vi "Trial 4 A4.vi"() -> ()   [LabVIEW 2022 SP3]
uses:
  Documents/Control 1 Trial 3.ctl
panel:
  out "Time remaining":i32
  in  "Start":bool
  in  "Stop":bool
  in  "Washing Mode Menu":T1(ring)
  out "Washing Stage":string
  out "Washing Mode":string
  in  "On/Off":bool
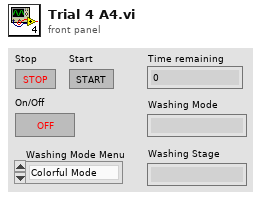
[diagram p1: front panel]
types:
  T1 = enum16{"Colorful Mode", "Intensive Mode", "Quick Wash"}
  T2 = typedef "Control 1 Trial 3.ctl" = enum16{"Off", "On", "Start Washing", "Pre-rinse", "Main Washing", "Final Spin", "Done Washing"}
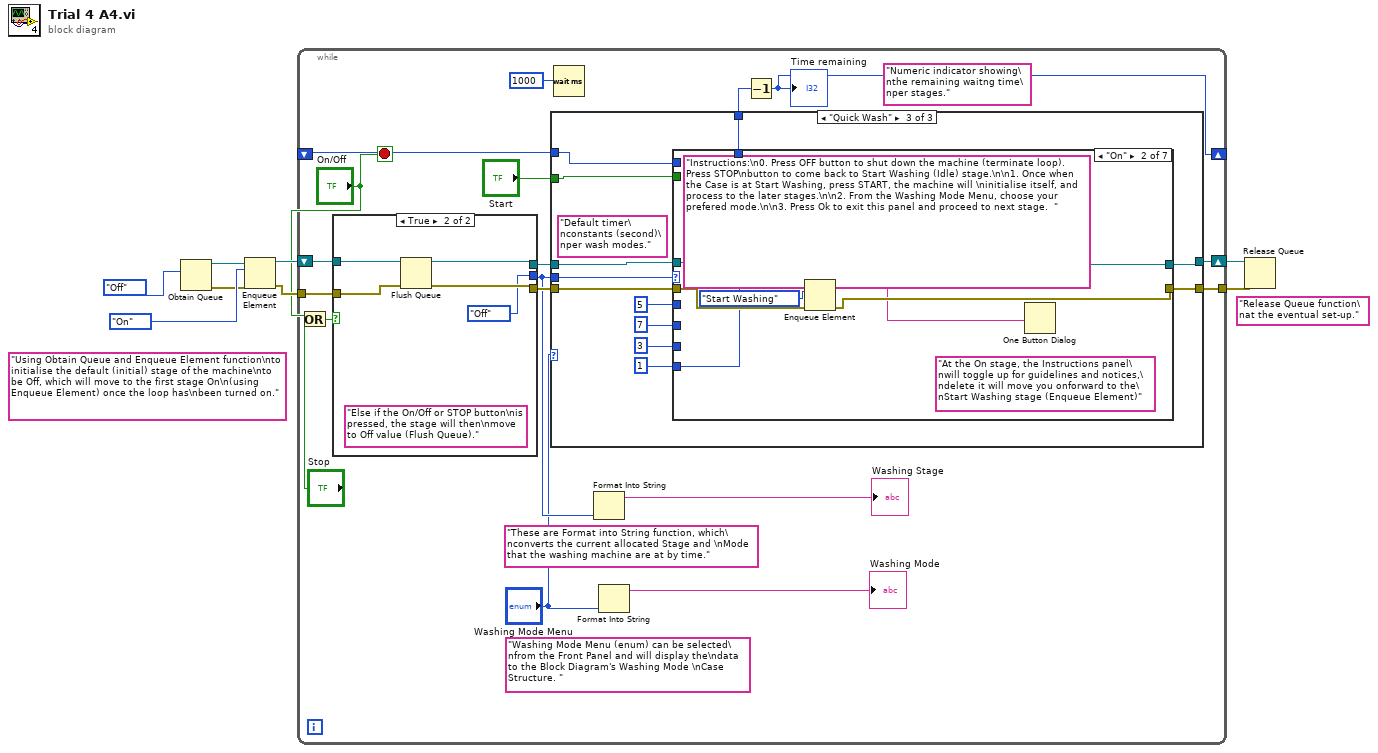
[diagram p0: block diagram]
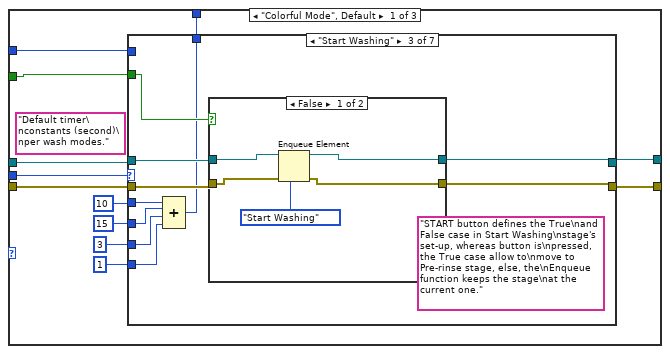
[diagram p2: hidden frame]
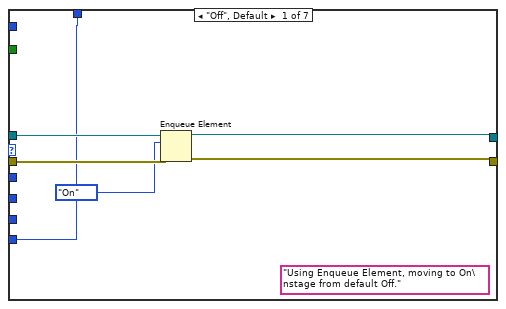
[diagram p3: hidden frame]
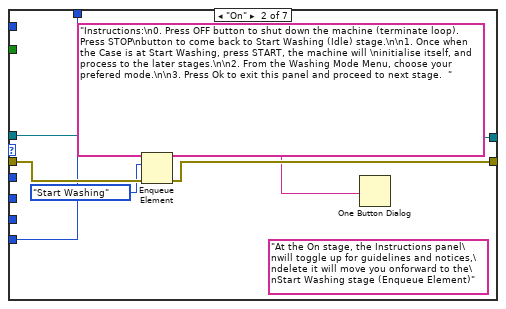
[diagram p4: hidden frame]
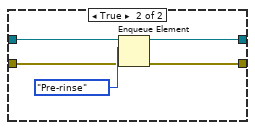
[diagram p5: hidden frame]
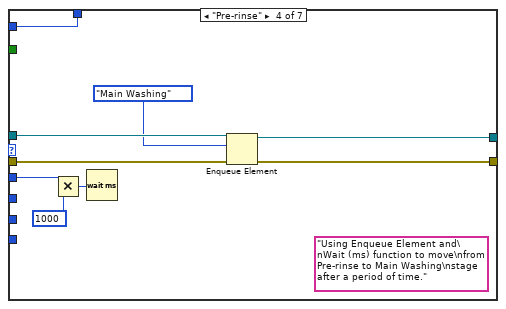
[diagram p6: hidden frame]
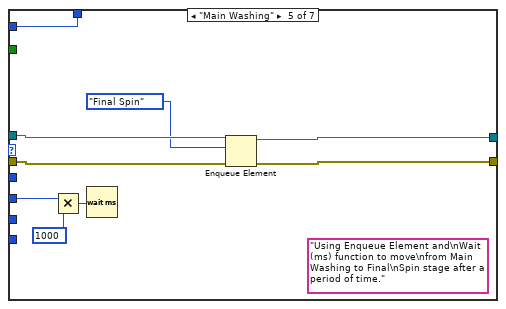
[diagram p7: hidden frame]
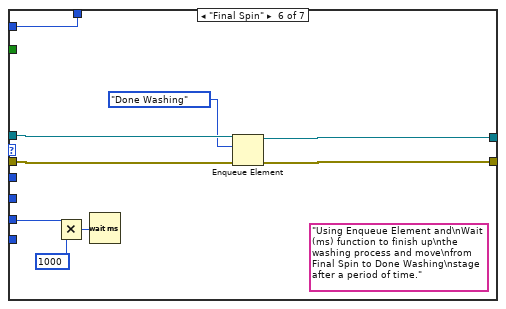
[diagram p8: hidden frame]
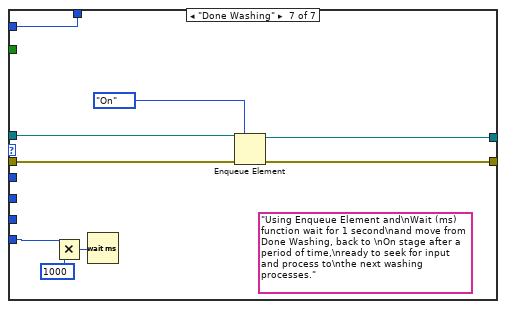
[diagram p9: hidden frame]
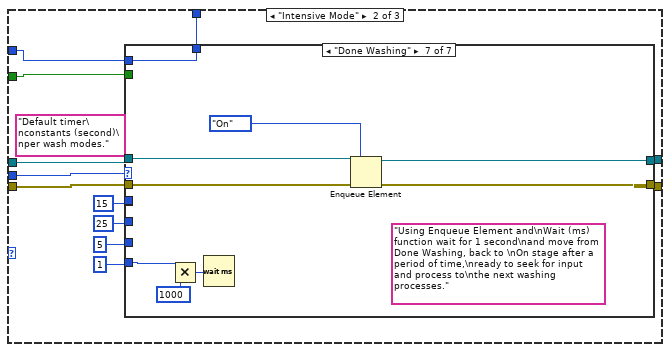
[diagram p10: hidden frame]
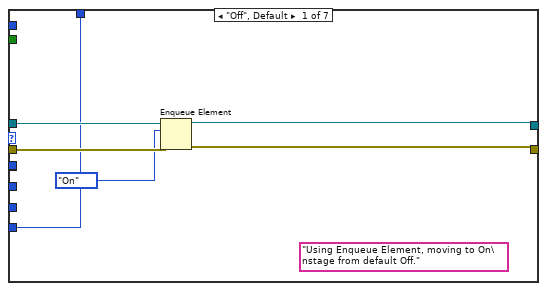
[diagram p11: hidden frame]
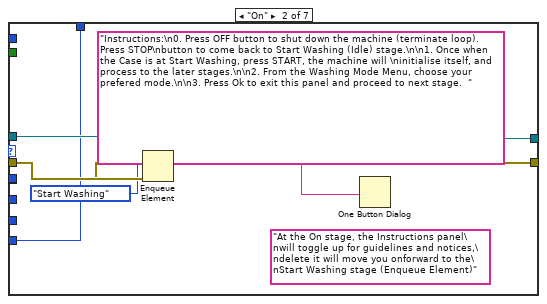
[diagram p12: hidden frame]
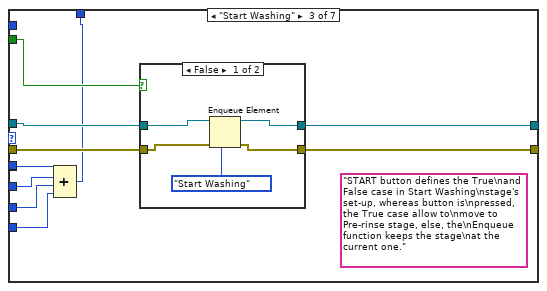
[diagram p13: hidden frame]
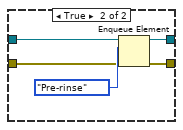
[diagram p14: hidden frame]
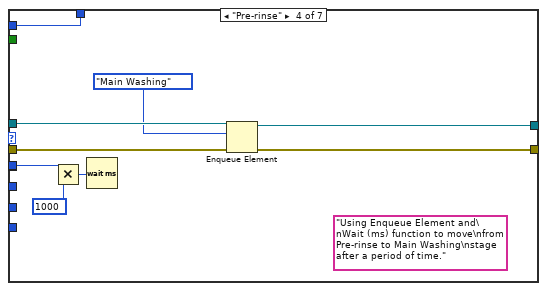
[diagram p15: hidden frame]
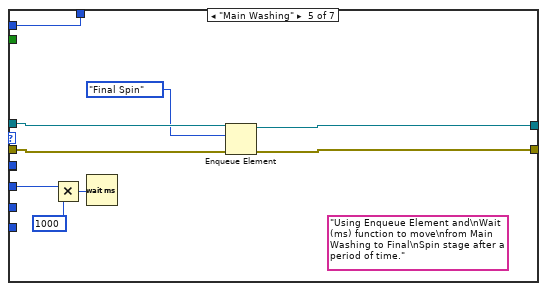
[diagram p16: hidden frame]
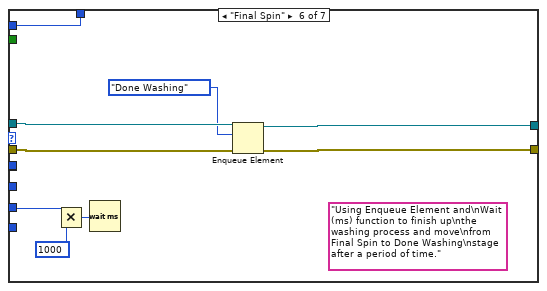
[diagram p17: hidden frame]
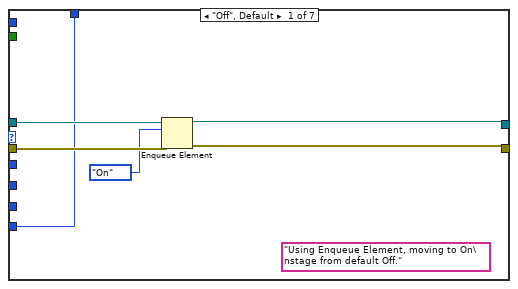
[diagram p18: hidden frame]
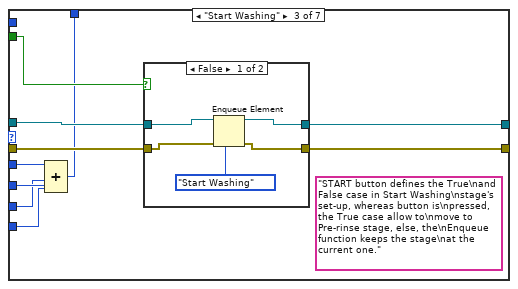
[diagram p19: hidden frame]
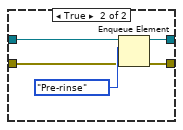
[diagram p20: hidden frame]
diagram:
  (unwired) "Release Queue function\nat the eventual set-up."
  (unwired) "Using Obtain Queue and Enqueue Element function\nto initialise the default (initial) stage of the machine\nto be Off, which will move to the first stage On\n(using Enqueue Element) once the loop has\nbeen turned on."
  n1 = Obtain Queue(element data type=Control_1_Trial_3."Off") -> (queue out=w8:refnum<queue>, error out=w2:errorcluster)  [unwired: 4 in, 1 out]
  n2 = Enqueue Element(queue=w8, element=Control_1_Trial_3."On", error in (no error)=w2) -> (queue out=w7:refnum<queue>, error out=w1:errorcluster)  [unwired: 1 in, 1 out]
  n3 = while {
    shift-right: [w20] -> w5
    shift-left: w7 -> [w25]
    tunnel: w1 -> [w26]
    tunnel: [w19] -> w6
    shift-right: [w12] -> _
    shift-left: _ -> [w13]
    stop <- "On/Off" stop-if-true
    (unwired) "Numeric indicator showing\nthe remaining waitng time\nper stages."
    (unwired) "Washing Mode Menu (enum) can be selected\nfrom the Front Panel and will display the\ndata to the Block Diagram's Washing Mode \nCase Structure. "
    (unwired) "These are Format into String function, which\nconverts the current allocated Stage and \nMode that the washing machine are at by time."
    n4 = Or(x="On/Off", y="Stop") -> (x .or. y?=w18:bool)
    n5 = case shown="True" w18 {
      tunnel: w26 -> [w273 w278]
      tunnel: w25 -> [w274 w279]
      tunnel: [w270 w276] -> w23
      tunnel: [w271 w277] -> w22
      tunnel: [w272 Control_1_Trial_3."Off"] -> w17
      frame False {
        (unwired) "If the On/Off or STOP button\nis not pressed, the stage will\nremains at the original On value\n(Dequeue Element)."
        n6 = Dequeue Element(queue=w274, error in (no error)=w273) -> (queue out=w270:refnum<queue>, element=w272:T2, error out=w271:errorcluster)  [unwired: 1 in, 1 out]
      }
      frame True {
        (unwired) "Else if the On/Off or STOP button\nis  pressed, the stage will then\nmove to Off value (Flush Queue)."
        n7 = Flush Queue(queue=w279, error in (no error)=w278) -> (queue out=w276:refnum<queue>, error out=w277:errorcluster)  [unwired: 1 out]
      }
    }
    n8 = case shown="\"Quick Wash\"" "Washing Mode Menu" {
      tunnel: w23 -> [w38 w119 w200]
      tunnel: [w35 w118 w198] -> w20
      tunnel: w22 -> [w37 w117 w199]
      tunnel: [w34 w116 w192] -> w19
      tunnel: w17 -> [w36 w115 w193]
      tunnel: "Start" -> [w29 w110 w191]
      tunnel: w13 -> [w27 w108 w190]
      tunnel: [w28 w109 w189] -> w11
      frame "Colorful Mode", Default {
        (unwired) "Default timer\nconstants (second)\nper wash modes."
        n9 = case shown="\"Start Washing\"" w36 {
          tunnel: w38 -> [w44 w51 w61 w80 w89 w98 w105]
          tunnel: [w41 w50 w59 w78 w87 w96 w107] -> w35
          tunnel: w37 -> [w43 w49 w60 w79 w88 w97 w104]
          tunnel: [w42 w48 w58 w77 w86 w95 w106] -> w34
          tunnel: 15 -> [_ _ w55 _ w82 _ _]
          tunnel: 3 -> [_ _ w54 _ _ w91 _]
          tunnel: 1 -> [w39 w45 w53 _ _ _ w100]
          tunnel: 10 -> [_ _ w56 w75 _ _ _]
          tunnel: w29 -> [_ _ w57 _ _ _ _]
          tunnel: w27 -> [_ _ _ w72 w81 w90 w99]
          tunnel: [w39 w45 w52 w72 w81 w90 w99] -> w28
          frame "Off", Default {
            (unwired) "Using Enqueue Element, moving to On\nstage from default Off."
            n10 = Enqueue Element(queue=w44, element=Control_1_Trial_3."On", error in (no error)=w43) -> (queue out=w41:refnum<queue>, error out=w42:errorcluster)  [unwired: 1 in, 1 out]
          }
          frame "On" {
            (unwired) "At the On stage, the Instructions panel\nwill toggle up for guidelines and notices,\ndelete it will move you onforward to the\nStart Washing stage (Enqueue Element)"
            n11 = Enqueue Element(queue=w51, element=Control_1_Trial_3."Start Washing", error in (no error)=w49) -> (queue out=w50:refnum<queue>, error out=w48:errorcluster)  [unwired: 1 in, 1 out]
            n12 = One Button Dialog(message="Instructions:\n0. Press OFF button to shut down the machine (terminate loop). Press STOP\nbutton to come back to Start Washing (Idle) stage.\n\n1. Once when the Case is at Start Washing, press START, the machine will \ninitialise itself, and process to the later stages.\n\n2. From the Washing Mode Menu, choose your prefered mode.\n\n3. Press Ok to exit this panel and proceed to next stage.  ") -> ()  [unwired: 1 in, 1 out]
          }
          frame "Start Washing" {
            (unwired) "START button defines the True\nand False case in Start Washing\nstage's set-up, whereas button is\npressed, the True case allow to\nmove to Pre-rinse stage, else, the\nEnqueue function keeps the stage\nat the current one."
            n13 = Compound Arithmetic op=unknown(w56, w55, w54, w53) -> (w52:i32)
            n14 = case shown="False" w57 {
              tunnel: w61 -> [w66 w71]
              tunnel: w60 -> [w65 w69]
              tunnel: [w63 w68] -> w59
              tunnel: [w64 w67] -> w58
              frame False {
                n15 = Enqueue Element(queue=w66, element=Control_1_Trial_3."Start Washing", error in (no error)=w65) -> (queue out=w63:refnum<queue>, error out=w64:errorcluster)  [unwired: 1 in, 1 out]
              }
              frame True {
                n16 = Enqueue Element(queue=w71, element=Control_1_Trial_3."Pre-rinse", error in (no error)=w69) -> (queue out=w68:refnum<queue>, error out=w67:errorcluster)  [unwired: 1 in, 1 out]
              }
            }
          }
          frame "Pre-rinse" {
            (unwired) "Using Enqueue Element and\nWait (ms) function to move\nfrom Pre-rinse to Main Washing\nstage after a period of time."
            n17 = Multiply(x=w75, y=1000) -> (x*y=w73:i32)
            n18 = Wait (ms)(milliseconds to wait=w73) -> ()  [unwired: 1 out]
            n19 = Enqueue Element(queue=w80, element=Control_1_Trial_3."Main Washing", error in (no error)=w79) -> (queue out=w78:refnum<queue>, error out=w77:errorcluster)  [unwired: 1 in, 1 out]
          }
          frame "Main Washing" {
            (unwired) "Using Enqueue Element and\nWait (ms) function to move\nfrom Main Washing to Final\nSpin stage after a period of time."
            n20 = Multiply(x=w82, y=1000) -> (x*y=w83:i32)
            n21 = Wait (ms)(milliseconds to wait=w83) -> ()  [unwired: 1 out]
            n22 = Enqueue Element(queue=w89, element=Control_1_Trial_3."Final Spin", error in (no error)=w88) -> (queue out=w87:refnum<queue>, error out=w86:errorcluster)  [unwired: 1 in, 1 out]
          }
          frame "Final Spin" {
            (unwired) "Using Enqueue Element and\nWait (ms) function to finish up\nthe washing process and move\nfrom Final Spin to Done Washing\nstage after a period of time."
            n23 = Multiply(x=w91, y=1000) -> (x*y=w92:i32)
            n24 = Wait (ms)(milliseconds to wait=w92) -> ()  [unwired: 1 out]
            n25 = Enqueue Element(queue=w98, element=Control_1_Trial_3."Done Washing", error in (no error)=w97) -> (queue out=w96:refnum<queue>, error out=w95:errorcluster)  [unwired: 1 in, 1 out]
          }
          frame "Done Washing" {
            (unwired) "Using Enqueue Element and\nWait (ms) function wait for 1 second\nand move from Done Washing, back to \nOn stage after a period of time,\nready to seek for input and process to\nthe next washing processes."
            n26 = Multiply(x=w100, y=1000) -> (x*y=w101:i32)
            n27 = Wait (ms)(milliseconds to wait=w101) -> ()  [unwired: 1 out]
            n28 = Enqueue Element(queue=w105, element=Control_1_Trial_3."On", error in (no error)=w104) -> (queue out=w107:refnum<queue>, error out=w106:errorcluster)  [unwired: 1 in, 1 out]
          }
        }
      }
      frame "Intensive Mode" {
        (unwired) "Default timer\nconstants (second)\nper wash modes."
        w111 = 15
        n29 = case shown="\"Done Washing\"" w115 {
          tunnel: w119 -> [w125 w132 w140 w161 w170 w179 w186]
          tunnel: [w122 w131 w142 w159 w168 w177 w188] -> w118
          tunnel: w117 -> [w124 w130 w139 w160 w169 w178 w185]
          tunnel: [w123 w129 w141 w158 w167 w176 w187] -> w116
          tunnel: w111 -> [_ _ w137 _ _ _ _]
          tunnel: 25 -> [_ _ w136 _ w163 _ _]
          tunnel: 5 -> [_ _ w135 _ _ w172 _]
          tunnel: 1 -> [w120 w126 w134 _ _ _ w181]
          tunnel: w111 -> [_ _ _ w156 _ _ _]
          tunnel: w110 -> [_ _ w138 _ _ _ _]
          tunnel: w108 -> [_ _ _ w153 w162 w171 w180]
          tunnel: [w120 w126 w133 w153 w162 w171 w180] -> w109
          frame "Off", Default {
            (unwired) "Using Enqueue Element, moving to On\nstage from default Off."
            n30 = Enqueue Element(queue=w125, element=Control_1_Trial_3."On", error in (no error)=w124) -> (queue out=w122:refnum<queue>, error out=w123:errorcluster)  [unwired: 1 in, 1 out]
          }
          frame "On" {
            (unwired) "At the On stage, the Instructions panel\nwill toggle up for guidelines and notices,\ndelete it will move you onforward to the\nStart Washing stage (Enqueue Element)"
            n31 = Enqueue Element(queue=w132, element=Control_1_Trial_3."Start Washing", error in (no error)=w130) -> (queue out=w131:refnum<queue>, error out=w129:errorcluster)  [unwired: 1 in, 1 out]
            n32 = One Button Dialog(message="Instructions:\n0. Press OFF button to shut down the machine (terminate loop). Press STOP\nbutton to come back to Start Washing (Idle) stage.\n\n1. Once when the Case is at Start Washing, press START, the machine will \ninitialise itself, and process to the later stages.\n\n2. From the Washing Mode Menu, choose your prefered mode.\n\n3. Press Ok to exit this panel and proceed to next stage.  ") -> ()  [unwired: 1 in, 1 out]
          }
          frame "Start Washing" {
            (unwired) "START button defines the True\nand False case in Start Washing\nstage's set-up, whereas button is\npressed, the True case allow to\nmove to Pre-rinse stage, else, the\nEnqueue function keeps the stage\nat the current one."
            n33 = Compound Arithmetic op=unknown(w137, w136, w135, w134) -> (w133:i32)
            n34 = case shown="False" w138 {
              tunnel: w140 -> [w147 w152]
              tunnel: w139 -> [w146 w150]
              tunnel: [w144 w149] -> w142
              tunnel: [w145 w148] -> w141
              frame False {
                n35 = Enqueue Element(queue=w147, element=Control_1_Trial_3."Start Washing", error in (no error)=w146) -> (queue out=w144:refnum<queue>, error out=w145:errorcluster)  [unwired: 1 in, 1 out]
              }
              frame True {
                n36 = Enqueue Element(queue=w152, element=Control_1_Trial_3."Pre-rinse", error in (no error)=w150) -> (queue out=w149:refnum<queue>, error out=w148:errorcluster)  [unwired: 1 in, 1 out]
              }
            }
          }
          frame "Pre-rinse" {
            (unwired) "Using Enqueue Element and\nWait (ms) function to move\nfrom Pre-rinse to Main Washing\nstage after a period of time."
            n37 = Multiply(x=w156, y=1000) -> (x*y=w154:i32)
            n38 = Wait (ms)(milliseconds to wait=w154) -> ()  [unwired: 1 out]
            n39 = Enqueue Element(queue=w161, element=Control_1_Trial_3."Main Washing", error in (no error)=w160) -> (queue out=w159:refnum<queue>, error out=w158:errorcluster)  [unwired: 1 in, 1 out]
          }
          frame "Main Washing" {
            (unwired) "Using Enqueue Element and\nWait (ms) function to move\nfrom Main Washing to Final\nSpin stage after a period of time."
            n40 = Multiply(x=w163, y=1000) -> (x*y=w164:i32)
            n41 = Wait (ms)(milliseconds to wait=w164) -> ()  [unwired: 1 out]
            n42 = Enqueue Element(queue=w170, element=Control_1_Trial_3."Final Spin", error in (no error)=w169) -> (queue out=w168:refnum<queue>, error out=w167:errorcluster)  [unwired: 1 in, 1 out]
          }
          frame "Final Spin" {
            (unwired) "Using Enqueue Element and\nWait (ms) function to finish up\nthe washing process and move\nfrom Final Spin to Done Washing\nstage after a period of time."
            n43 = Multiply(x=w172, y=1000) -> (x*y=w173:i32)
            n44 = Wait (ms)(milliseconds to wait=w173) -> ()  [unwired: 1 out]
            n45 = Enqueue Element(queue=w179, element=Control_1_Trial_3."Done Washing", error in (no error)=w178) -> (queue out=w177:refnum<queue>, error out=w176:errorcluster)  [unwired: 1 in, 1 out]
          }
          frame "Done Washing" {
            (unwired) "Using Enqueue Element and\nWait (ms) function wait for 1 second\nand move from Done Washing, back to \nOn stage after a period of time,\nready to seek for input and process to\nthe next washing processes."
            n46 = Multiply(x=w181, y=1000) -> (x*y=w182:i32)
            n47 = Wait (ms)(milliseconds to wait=w182) -> ()  [unwired: 1 out]
            n48 = Enqueue Element(queue=w186, element=Control_1_Trial_3."On", error in (no error)=w185) -> (queue out=w188:refnum<queue>, error out=w187:errorcluster)  [unwired: 1 in, 1 out]
          }
        }
      }
      frame "Quick Wash" {
        (unwired) "Default timer\nconstants (second)\nper wash modes."
        n49 = case shown="\"On\"" w193 {
          tunnel: w200 -> [w206 w213 w223 w242 w251 w260 w267]
          tunnel: [w204 w212 w221 w240 w249 w258 w269] -> w198
          tunnel: w199 -> [w203 w211 w222 w241 w250 w259 w266]
          tunnel: [w205 w210 w220 w239 w248 w257 w268] -> w192
          tunnel: 7 -> [_ _ w217 _ w244 _ _]
          tunnel: 3 -> [_ _ w216 _ _ w253 _]
          tunnel: 1 -> [w201 w207 w215 _ _ _ w262]
          tunnel: 5 -> [_ _ w218 w235 _ _ _]
          tunnel: w191 -> [_ _ w219 _ _ _ _]
          tunnel: w190 -> [_ _ _ w234 w243 w252 w261]
          tunnel: [w201 w207 w214 w234 w243 w252 w261] -> w189
          frame "Off", Default {
            (unwired) "Using Enqueue Element, moving to On\nstage from default Off."
            n50 = Enqueue Element(queue=w206, element=Control_1_Trial_3."On", error in (no error)=w203) -> (queue out=w204:refnum<queue>, error out=w205:errorcluster)  [unwired: 1 in, 1 out]
          }
          frame "On" {
            (unwired) "At the On stage, the Instructions panel\nwill toggle up for guidelines and notices,\ndelete it will move you onforward to the\nStart Washing stage (Enqueue Element)"
            n51 = Enqueue Element(queue=w213, element=Control_1_Trial_3."Start Washing", error in (no error)=w211) -> (queue out=w212:refnum<queue>, error out=w210:errorcluster)  [unwired: 1 in, 1 out]
            n52 = One Button Dialog(message="Instructions:\n0. Press OFF button to shut down the machine (terminate loop). Press STOP\nbutton to come back to Start Washing (Idle) stage.\n\n1. Once when the Case is at Start Washing, press START, the machine will \ninitialise itself, and process to the later stages.\n\n2. From the Washing Mode Menu, choose your prefered mode.\n\n3. Press Ok to exit this panel and proceed to next stage.  ") -> ()  [unwired: 1 in, 1 out]
          }
          frame "Start Washing" {
            (unwired) "START button defines the True\nand False case in Start Washing\nstage's set-up, whereas button is\npressed, the True case allow to\nmove to Pre-rinse stage, else, the\nEnqueue function keeps the stage\nat the current one."
            n53 = Compound Arithmetic op=unknown(w218, w217, w216, w215) -> (w214:i32)
            n54 = case shown="False" w219 {
              tunnel: w223 -> [w228 w233]
              tunnel: w222 -> [w227 w231]
              tunnel: [w225 w230] -> w221
              tunnel: [w226 w229] -> w220
              frame False {
                n55 = Enqueue Element(queue=w228, element=Control_1_Trial_3."Start Washing", error in (no error)=w227) -> (queue out=w225:refnum<queue>, error out=w226:errorcluster)  [unwired: 1 in, 1 out]
              }
              frame True {
                n56 = Enqueue Element(queue=w233, element=Control_1_Trial_3."Pre-rinse", error in (no error)=w231) -> (queue out=w230:refnum<queue>, error out=w229:errorcluster)  [unwired: 1 in, 1 out]
              }
            }
          }
          frame "Pre-rinse" {
            (unwired) "Using Enqueue Element and\nWait (ms) function to move\nfrom Pre-rinse to Main Washing\nstage after a period of time."
            n57 = Multiply(x=w235, y=1000) -> (x*y=w236:i32)
            n58 = Wait (ms)(milliseconds to wait=w236) -> ()  [unwired: 1 out]
            n59 = Enqueue Element(queue=w242, element=Control_1_Trial_3."Main Washing", error in (no error)=w241) -> (queue out=w240:refnum<queue>, error out=w239:errorcluster)  [unwired: 1 in, 1 out]
          }
          frame "Main Washing" {
            (unwired) "Using Enqueue Element and\nWait (ms) function to move\nfrom Main Washing to Final\nSpin stage after a period of time."
            n60 = Multiply(x=w244, y=1000) -> (x*y=w245:i32)
            n61 = Wait (ms)(milliseconds to wait=w245) -> ()  [unwired: 1 out]
            n62 = Enqueue Element(queue=w251, element=Control_1_Trial_3."Final Spin", error in (no error)=w250) -> (queue out=w249:refnum<queue>, error out=w248:errorcluster)  [unwired: 1 in, 1 out]
          }
          frame "Final Spin" {
            (unwired) "Using Enqueue Element and\nWait (ms) function to finish up\nthe washing process and move\nfrom Final Spin to Done Washing\nstage after a period of time."
            n63 = Multiply(x=w253, y=1000) -> (x*y=w254:i32)
            n64 = Wait (ms)(milliseconds to wait=w254) -> ()  [unwired: 1 out]
            n65 = Enqueue Element(queue=w260, element=Control_1_Trial_3."Done Washing", error in (no error)=w259) -> (queue out=w258:refnum<queue>, error out=w257:errorcluster)  [unwired: 1 in, 1 out]
          }
          frame "Done Washing" {
            (unwired) "Using Enqueue Element and\nWait (ms) function wait for 1 second\nand move from Done Washing, back to \nOn stage after a period of time,\nready to seek for input and process to\nthe next washing processes."
            n66 = Multiply(x=w262, y=1000) -> (x*y=w263:i32)
            n67 = Wait (ms)(milliseconds to wait=w263) -> ()  [unwired: 1 out]
            n68 = Enqueue Element(queue=w267, element=Control_1_Trial_3."On", error in (no error)=w266) -> (queue out=w269:refnum<queue>, error out=w268:errorcluster)  [unwired: 1 in, 1 out]
          }
        }
      }
    }
    n69 = Wait (ms)(milliseconds to wait=1000) -> ()  [unwired: 1 out]
    n70 = Format Into String(w17) -> (resulting string=→"Washing Stage":string)  [unwired: 3 in, 1 out]
    n71 = Format Into String("Washing Mode Menu") -> (resulting string=→"Washing Mode":string)  [unwired: 3 in, 1 out]
    n72 = Decrement(x=w11) -> (x-1=w12:i32)
    "Time remaining" <- w12
  }
  n73 = Release Queue(queue=w5, error in (no error)=w6) -> ()  [unwired: 1 in, 3 out]
